vi "Get Tovey Data.vi"(11 "Model in":refnum<class "Model.lvclass">) -> (2 "ToveyData":T1[](array[typedef]) {"Timestamp" format="%.4f"; "Mz" format="%.4f"; "My" format="%.4f"; "Mx" format="%.4f"; "Fz" format="%.4f"; "Fy" format="%.4f"; "Fx" format="%.4f"}, 3 "Model out":refnum<class "Model.lvclass">)   [LabVIEW 2016]
uses:
  Model.lvclass
  Typedefs/ToveyEngData.ctl
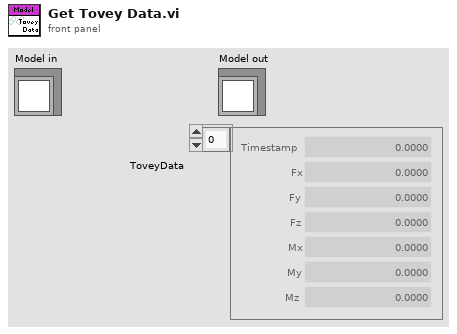
[diagram p1: front panel]
types:
  T1 = typedef "ToveyEngData.ctl" = cluster{"Timestamp":dbl, "Fx":dbl, "Fy":dbl, "Fz":dbl, "Mx":dbl, "My":dbl, "Mz":dbl}
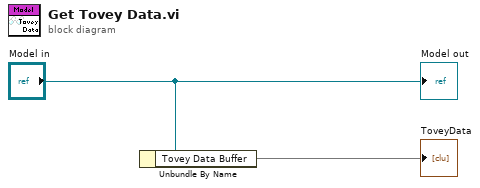
[diagram p0: block diagram]
diagram:
  n1 = Unbundle By Name("Model in") -> ("Tovey Data Buffer"=→"ToveyData")
  "Model out" <- "Model in"
